vi "U3 eAIN Example.vi"() -> (0 "error out":errorcluster)   [LabVIEW 2021]
panel:
  in  "Binary":bool
  in  "ChannelN":i32=31
  in  "ChannelP":i32
  in  "FirstFound":bool=TRUE
  in  "Address":string="1"
  out "Error Message":string
  out "Value Read":dbl format="%.6f"
  # "Reads 1 analog input using the UD easy function eAIN."
  # "30 = Temp Sensor\n31 = Vreg"
  # "30 = Vref\n31 = Single Ended\n32 = Special 0-3.6"
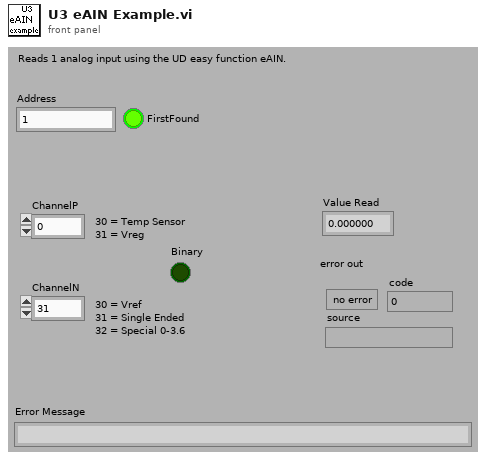
[diagram p1: front panel]
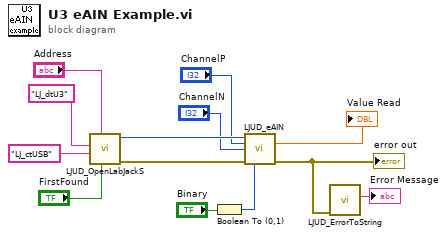
[diagram p0: block diagram]
diagram:
  n1 = call "LJUD_OpenLabJackS.vi"("FirstFound"="FirstFound", "Address"="Address", "ConnectionType"="LJ_ctUSB", "DeviceType"="LJ_dtU3") -> ("error out"=w7:errorcluster, "Handle"=w8:i32)  [unwired: 5 in, 1 out]
  n2 = Boolean To (0,1)(Boolean="Binary") -> (0, 1=w1:i16)
  n3 = call "LJUD_eAIN.vi"("Handle In"=w8, "ChannelP"="ChannelP", "ChannelN"="ChannelN", "error in"=w7, "Binary"=w1) -> ("Voltage"=→"Value Read":dbl, "error out"=w6:errorcluster)  [unwired: 8 in, 1 out]
  "error out" <- w6
  n4 = call "LJUD_ErrorToString.vi"("error in"=w6) -> ("String"=→"Error Message":string)  [unwired: 10 in]
